vi "UDP Heartbeat Transmitter.vi"(0 "Interval Length":i32, 1 "connection ID":refnum<k16>, 2 "Remote UDP Address":u32, 3 "Remote UDP Port":i32, 7 "Count":i32, 11 "error in (no error)":errorcluster) -> (15 "error out":errorcluster)   [LabVIEW 2013]
uses:
  UDP Heartbeat Globals.vi
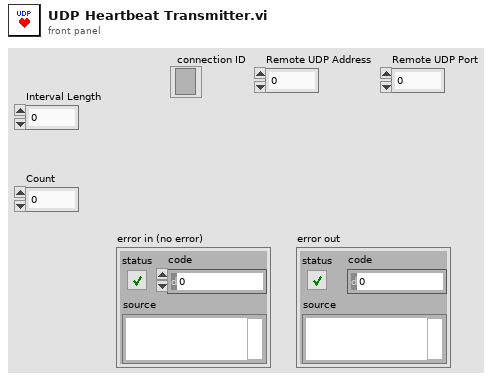
[diagram p1: front panel]
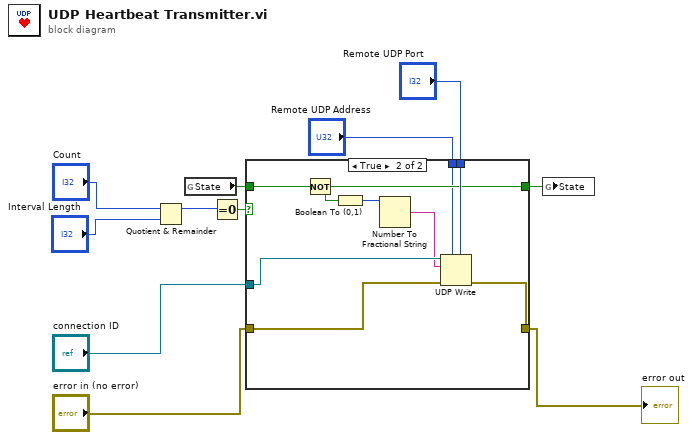
[diagram p0: block diagram]
diagram:
  n1 = Quotient & Remainder(x="Count", y="Interval Length") -> (x-y*floor(x/y)=w9:i32)  [unwired: 1 out]
  n2 = global read "UDP Heartbeat Globals.vi" "State"() -> (w6:bool)
  n3 = Equal To 0?(x=w9) -> (x = 0?=w8:bool)
  n4 = case shown="True" w8 {
    tunnel: w6 -> [w13 w22]
    tunnel: [w13 w18] -> w7
    tunnel: "Remote UDP Port" -> [_ w21]
    tunnel: "connection ID" -> [_ w20]
    tunnel: "error in (no error)" -> [w12 w19]
    tunnel: [w12 w15] -> w2
    tunnel: "Remote UDP Address" -> [_ w14]
    frame False {
    }
    frame True {
      n5 = Not(x=w22) -> (.not. x?=w18:bool)
      n6 = Boolean To (0,1)(Boolean=w18) -> (0, 1=w17:i16)
      n7 = Number To Fractional String(number=w17) -> (F-format string=w16:string)  [unwired: 3 in]
      n8 = UDP Write(address=w14, port or service name=w21, connection ID=w20, data in=w16, 8:w19) -> (error out=w15:errorcluster)  [unwired: 1 in, 1 out]
    }
  }
  "error out" <- w2
  n9 = global write "UDP Heartbeat Globals.vi" "State"(w7) -> ()
